vi "Vision Processing.vi"(4 "error in (no error)":errorcluster, 7 "Image Size":T1=enum."320x240") -> ()   [LabVIEW 2018]
doc: "This VI runs in parallel to other tasks. It gets images from the camera, processes them for color or shape and use that information to affect robot behavior."
uses:
  <vilib>/Rock Robotics/WPI/Camera/WPI_CameraImageSize.ctl
  <vilib>/Rock Robotics/WPI/Camera/WPI_CameraWhite Balance Values.ctl
  <vilib>/Rock Robotics/WPI/Camera/WPI_CameraExposure Values.ctl
  <vilib>/Rock Robotics/WPI/Camera/WPI_CameraFrameRate.ctl
panel:
  in  "Image Size 2":T1=enum."320x240"
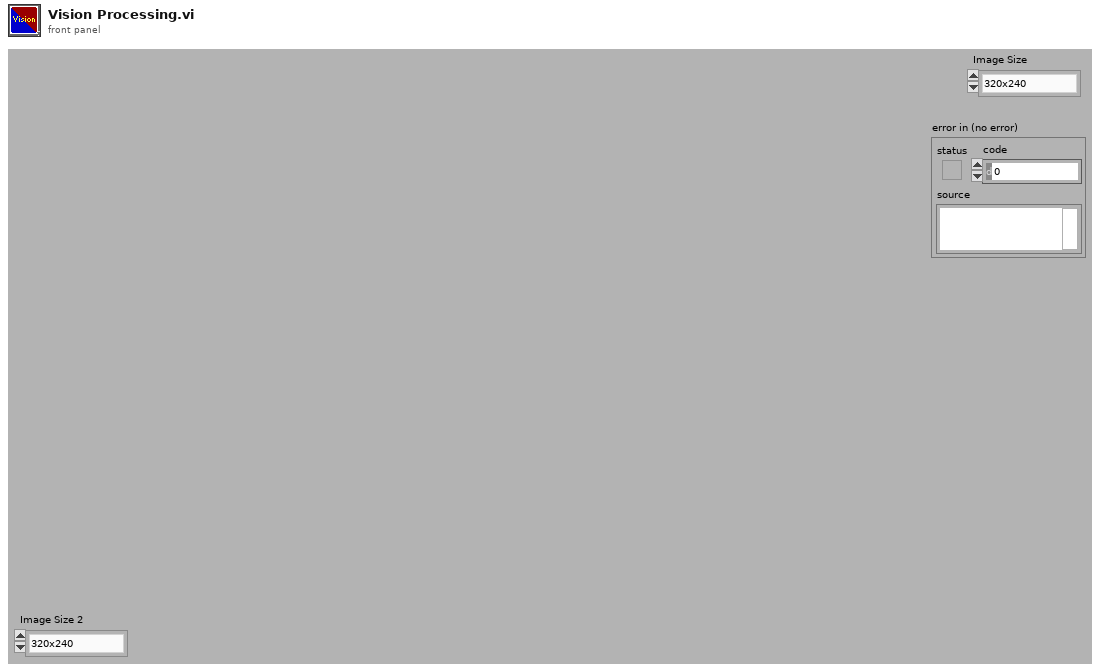
[diagram p1: front panel]
types:
  T1 = typedef "WPI_CameraImageSize.ctl" = enum16{"640x480", "320x240", "160x120", "Custom"}
  T2 = typedef "WPI_CameraFrameRate.ctl" = u32
  T3 = typedef "WPI_CameraExposure Values.ctl" = enum16{"Auto", "Flicker-free 50 Hz", "Flicker-free 60 Hz", "Hold current", "Custom"}
  T4 = typedef "WPI_CameraWhite Balance Values.ctl" = enum16{"Auto", "Fixed indoor", "Fixed outdoor 1", "Fixed outdoor 2", "Fixed fluorescent 1", "Fixed fluorescent 2", "Hold current", "Custom"}
  T5 = typedef "Image Type" = u32
  T6 = typedef "WPI_CameraDevRef.ctl" = cluster{"Camera Address":string, "CameraStatus":errorcluster}
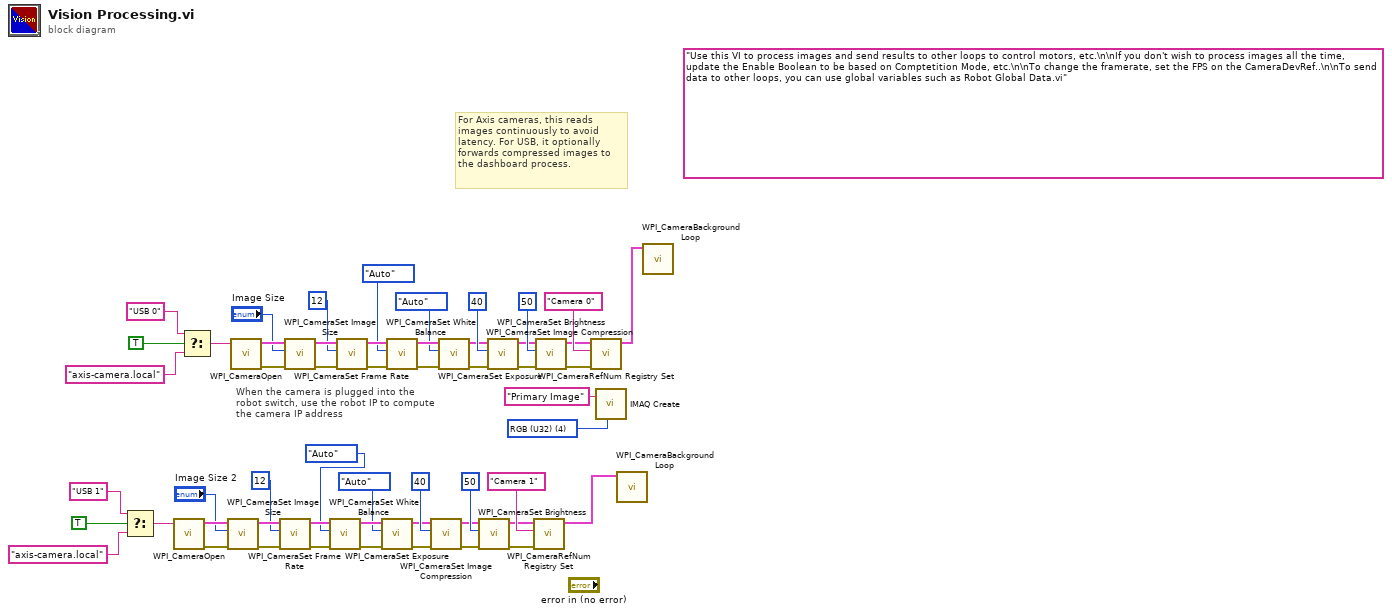
[diagram p0: block diagram]
diagram:
  (unwired) "Use this VI to process images and send results to other loops to control motors, etc.\n\nIf you don't wish to process images all the time, update the Enable Boolean to be based on Comptetition Mode, etc.\n\nTo change the framerate, set the FPS on the CameraDevRef..\n\nTo send data to other loops, you can use global variables such as Robot Global Data.vi"
  w54 = T5 4 items=["Grayscale (U8)", "Grayscale (I16)", "Grayscale (SGL)", "Complex (CSG)", "RGB (U32)", "HSL (U32)", "RGB (U64)"] ("Image Type")
  # "When the camera is plugged into the\nrobot switch, use the robot IP to compute\nthe camera IP address"
  # "For Axis cameras, this reads\nimages continuously to avoid\nlatency. For USB, it optionally\nforwards compressed images to\nthe dashboard process."
  n1 = Select(t="USB 1" ("format string"), s=TRUE ("dot notation? (F)"), f="axis-camera.local" ("format string")) -> (s? t:f=w4:string)
  n2 = call <vilib>:"WPI_CameraOpen.vi"("Camera Address"=w4) -> ("error out"=w17:errorcluster, "CameraDevRef"=w18:T6)  [unwired: 1 in, 8 out]
  n3 = Select(t="USB 0" ("format string"), s=TRUE ("dot notation? (F)"), f="axis-camera.local" ("format string")) -> (s? t:f=w28:string)
  n4 = call <vilib>:"WPI_CameraSet Image Size.vi"("error in (no error)"=w17, "Image Size"="Image Size 2", "CameraDevRef"=w18) -> ("error out"=w16:errorcluster, "CameraDevRef Out"=w19:T6)  [unwired: 1 in, 6 out]
  n5 = call <vilib>:"WPI_CameraOpen.vi"("Camera Address"=w28) -> ("error out"=w43:errorcluster, "CameraDevRef"=w44:T6)  [unwired: 1 in, 8 out]
  n6 = call <vilib>:"WPI_CameraSet Frame Rate.vi"("error in (no error)"=w16, "Frame Rate (fps)"=T2 12, "CameraDevRef"=w19) -> ("error out"=w15:errorcluster, "CameraDevRef Out"=w21:T6)  [unwired: 7 out]
  n7 = call <vilib>:"WPI_CameraSet Image Size.vi"("error in (no error)"=w43, "Image Size"="Image Size", "CameraDevRef"=w44) -> ("error out"=w42:errorcluster, "CameraDevRef Out"=w45:T6)  [unwired: 1 in, 6 out]
  n8 = call <vilib>:"WPI_CameraSet White Balance.vi"("error in (no error)"=w15, "White Balance"=WPI_CameraWhite_Balance_Values."Auto", "CameraDevRef"=w21) -> ("error out"=w14:errorcluster, "CameraDevRef Out"=w20:T6)  [unwired: 1 in, 6 out]
  n9 = call <vilib>:"WPI_CameraSet Frame Rate.vi"("error in (no error)"=w42, "Frame Rate (fps)"=T2 12, "CameraDevRef"=w45) -> ("error out"=w41:errorcluster, "CameraDevRef Out"=w47:T6)  [unwired: 7 out]
  n10 = call <vilib>:"WPI_CameraSet Exposure.vi"("error in (no error)"=w14, "Exposure"=WPI_CameraExposure_Values."Auto", "CameraDevRef"=w20) -> ("error out"=w13:errorcluster, "CameraDevRef Out"=w23:T6)  [unwired: 1 in, 6 out]
  n11 = call <vilib>:"WPI_CameraSet White Balance.vi"("error in (no error)"=w41, "White Balance"=WPI_CameraWhite_Balance_Values."Auto", "CameraDevRef"=w47) -> ("error out"=w40:errorcluster, "CameraDevRef Out"=w46:T6)  [unwired: 1 in, 6 out]
  n12 = call <vilib>:"WPI_CameraSet Image Compression.vi"("error in (no error)"=w13, "Compression"=40, "CameraDevRef"=w23) -> ("error out"=w12:errorcluster, "CameraDevRef Out"=w22:T6)  [unwired: 7 out]
  n13 = call <vilib>:"WPI_CameraSet Exposure.vi"("error in (no error)"=w40, "Exposure"=WPI_CameraExposure_Values."Auto", "CameraDevRef"=w46) -> ("error out"=w39:errorcluster, "CameraDevRef Out"=w49:T6)  [unwired: 1 in, 6 out]
  n14 = call <vilib>:"WPI_CameraSet Brightness.vi"("error in (no error)"=w12, "Brightness"=50, "CameraDevRef"=w22) -> ("error out"=w10:errorcluster, "CameraDevRef Out"=w11:T6)  [unwired: 1 in, 6 out]
  n15 = call <vilib>:"WPI_CameraSet Image Compression.vi"("error in (no error)"=w39, "Compression"=40, "CameraDevRef"=w49) -> ("error out"=w38:errorcluster, "CameraDevRef Out"=w48:T6)  [unwired: 7 out]
  n16 = call <vilib>:"WPI_CameraRefNum Registry Set.vi"("error in (no error)"=w10, "refnum name"="Camera 1", "CameraDevRef"=w11) -> ("CameraDevRef"=w1:T6)  [unwired: 1 in, 7 out]
  n17 = call <vilib>:"WPI_CameraSet Brightness.vi"("error in (no error)"=w38, "Brightness"=50, "CameraDevRef"=w48) -> ("error out"=w36:errorcluster, "CameraDevRef Out"=w37:T6)  [unwired: 1 in, 6 out]
  n18 = call <vilib>:"WPI_CameraRefNum Registry Set.vi"("error in (no error)"=w36, "refnum name"="Camera 0", "CameraDevRef"=w37) -> ("CameraDevRef"=w32:T6)  [unwired: 1 in, 7 out]
  n19 = call "IMAQ Create"("Image Name"="Primary Image", "Image Type"=w54) -> ()  [unwired: 2 in, 3 out]
  n20 = call <vilib>:"WPI_CameraBackground Loop.vi"("CameraDevRef"=w1) -> ()  [unwired: 11 in]
  n21 = call <vilib>:"WPI_CameraBackground Loop.vi"("CameraDevRef"=w32) -> ()  [unwired: 11 in]
